vi "動態調整圓形.vi"() -> ()   [LabVIEW 2019]
panel:
  in  "半徑":dbl(slide) scale=0.0..100.0
  in  "y座標":dbl(slide) scale=-100.0..100.0
  in  "x座標":dbl(slide) scale=-100.0..100.0
  out "XY Graph":cluster{dbl[], dbl[]}(graph)
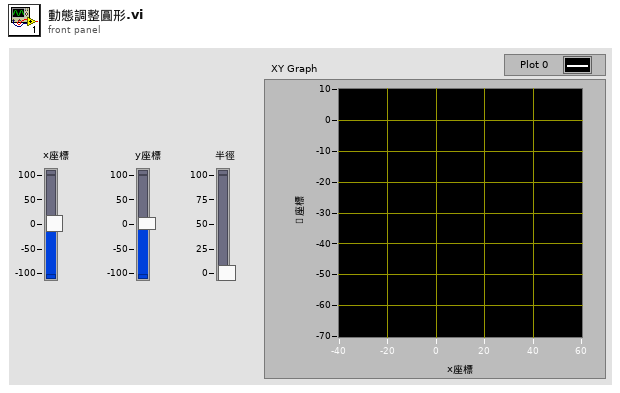
[diagram p1: front panel]
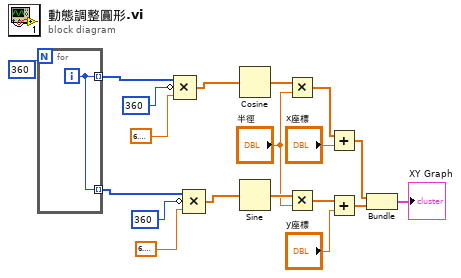
[diagram p0: block diagram]
diagram:
  n1 = for {
    N: 360 -> [_]
    tunnel: [w20] -> w8 mode=indexing
    tunnel: [w20] -> w4 mode=indexing
    i -> [w20]
  }
  n2 = Compound Arithmetic op=MULTIPLY(w8, invert 360, 6.283185307179586) -> (w6:dbl[])
  n3 = Compound Arithmetic op=MULTIPLY(w4, invert 360, 6.283185307179586) -> (w3:dbl[])
  n4 = Cosine(x=w6) -> (cos(x)=w15:dbl[])
  n5 = Sine(x=w3) -> (sin(x)=w17:dbl[])
  n6 = Multiply(x=w15, y="半徑") -> (x*y=w13:dbl[])
  n7 = Multiply(x=w17, y="半徑") -> (x*y=w16:dbl[])
  n8 = Add(x=w13, y="x座標") -> (x+y=w12:dbl[])
  n9 = Add(x=w16, y="y座標") -> (x+y=w11:dbl[])
  n10 = Bundle(w12, w11) -> (→"XY Graph":cluster{dbl[], dbl[]})  [unwired: 1 in]
